vi "PART_II.vi"() -> ()   [LabVIEW 2019]
uses:
  <vilib>/Analysis/baseanly.llb/Mean (DBL).vi
  <vilib>/Utility/file.llb/Read Delimited Spreadsheet (DBL).vi
  <vilib>/Analysis/NI_AALBase.lvlib
panel:
  out "Waveform Chart":dbl(graph)
  in  "n-point length":i32
  in  "time":dbl
  out "subarray":dbl[](array[numeric])
  out "all rows":dbl[][](array[numeric])
  in  "file path (dialog if empty)":path
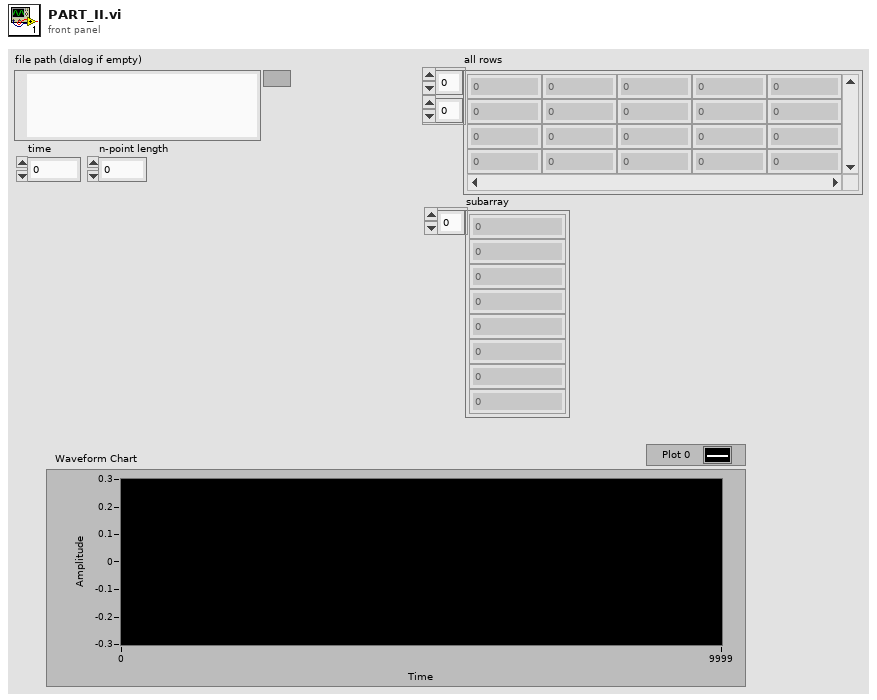
[diagram p1: front panel]
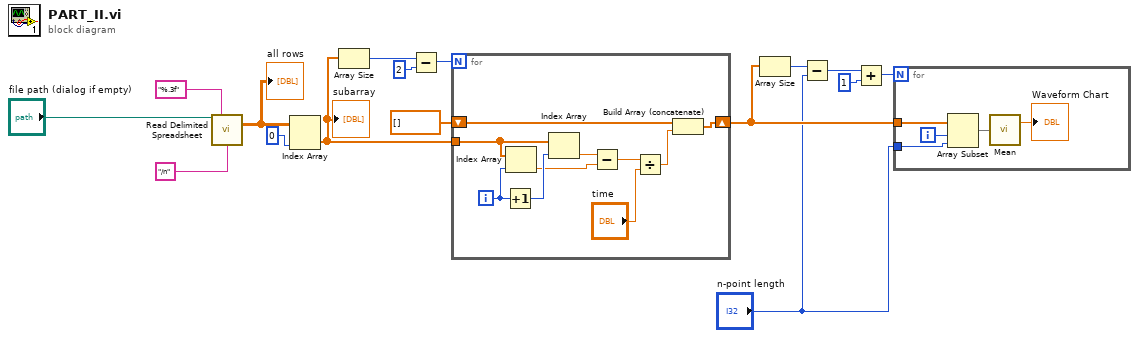
[diagram p0: block diagram]
diagram:
  n1 = call-poly <vilib>:"Read Delimited Spreadsheet.vi"("file path (dialog if empty)"="file path (dialog if empty)", "format (%.3f)"="%.3f", "delimiter (\\t)"="/n" ("delimiter (\\t)")) -> ("all rows"=w13:dbl[][])  [unwired: 7 in, 5 out]
  "all rows" <- w13
  n2 = Index Array(array=w13, index (col)=0 ("disabled index (col)")) -> (element=w10:dbl[])  [unwired: 1 in]
  "subarray" <- w10
  n3 = Array Size(array=w10) -> (size(s)=w9:i32)
  n4 = Subtract(x=w9, y=2) -> (x-y=w7:i32)
  n5 = for {
    N: w7 -> [_]
    tunnel: w10 -> [w24]
    shift-right: [w18] -> w6
    shift-left: dbl[] [] -> [w17]
    i -> [w25]
    n6 = Increment(x=w25) -> (x+1=w26:i32)
    n7 = Index Array(array=w24, index=w25) -> (element=w22:dbl)
    n8 = Index Array(array=w24, index=w26) -> (element=w23:dbl)
    n9 = Subtract(x=w23, y=w22) -> (x-y=w21:dbl)
    n10 = Divide(x=w21, y="time") -> (x/y=w19:dbl)
    n11 = Build Array (concatenate)(w17, w19) -> (w18:dbl[])
  }
  n12 = Array Size(array=w6) -> (size(s)=w5:i32)
  n13 = Subtract(x=w5, y="n-point length") -> (x-y=w3:i32)
  n14 = Add(x=w3, y=1) -> (x+y=w1:i32)
  n15 = for {
    N: w1 -> [_]
    tunnel: w6 -> [w31]
    tunnel: "n-point length" -> [w29]
    i -> [w30]
    n16 = Array Subset(array=w31, index=w30, length=w29) -> (w28:dbl[])
    n17 = call-poly <vilib>:"Mean.vi"("X"=w28) -> ("mean"=→"Waveform Chart":dbl)  [unwired: 1 out]
  }
